vi "prueba_modbus.vi"() -> ()   [LabVIEW 2021, in "Test_VIs.lvlib"]
uses:
  Test_VIs.lvlib
  <vilib>/Modbus/master/Modbus Master.lvclass
  <vilib>/Modbus/master/Create Master Instance (TCP).vi
panel:
  out "ComunicacionCRIO":bool
  out "coil values":bool[](array[boolean])
  in  "stop":bool
  out "element":u16
  out "element 2":u16
  out "element 3":u16
  out "Array":sgl[](array[numeric])
  in  "coil values 2":bool[](array[boolean])
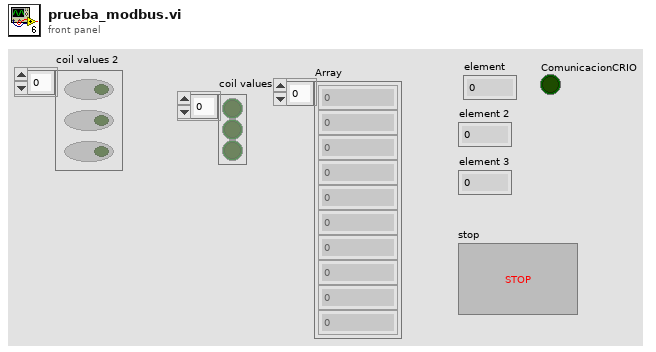
[diagram p1: front panel]
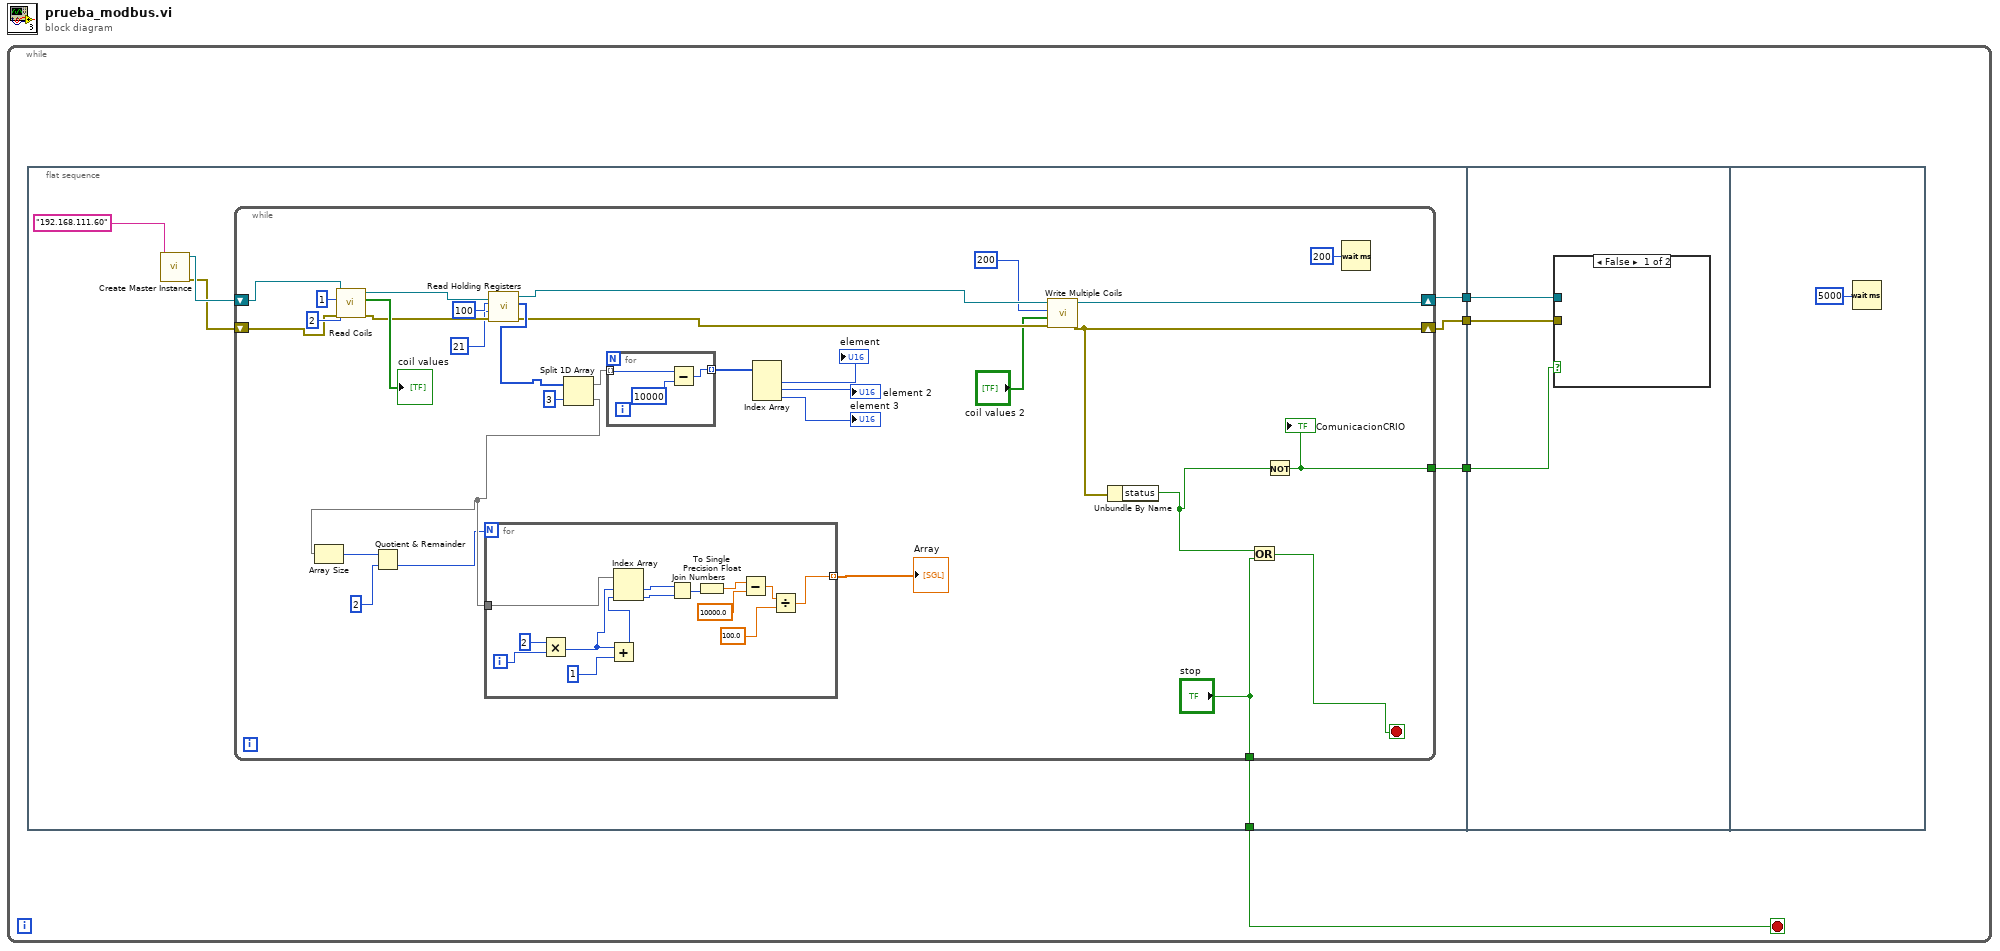
[diagram p0: block diagram]
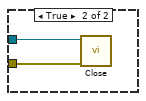
[diagram p2: hidden frame]
diagram:
  n1 = while {
    stop <- w1 stop-if-true
    n2 = flat-sequence {
      tunnel: [w8] -> w4
      tunnel: [w7] -> w3
      tunnel: [w6] -> w2
      tunnel: [w5] -> w1
      tunnel: w4 -> [w63]
      tunnel: w3 -> [w62]
      tunnel: w2 -> [w61]
      frame #0 {
        n3 = call-poly <vilib>:"Create Master Instance.vi"("address"="192.168.111.60") -> ("error out"=w9:errorcluster, "TCP master instance"=w10:refnum<class "Modbus Master.lvclass">)  [unwired: 9 in]
        n4 = while {
          shift-right: [w18] -> w7
          shift-left: w10 -> [w20]
          shift-right: [w17] -> w6
          shift-left: w9 -> [w19]
          tunnel: [w14] -> w8
          tunnel: ["stop"] -> w5
          stop <- w16 stop-if-true
          n5 = call-dynamic "Read Coils.vi"("error in (no error)"=w19, "number of coils"=u16 2, "starting address"=u16 1, "Modbus master in"=w20) -> ("error out"=w39:errorcluster, "coil values"=→"coil values":bool[], "Modbus master out"=w40:refnum<class "Modbus Master.lvclass">)  [unwired: 5 in]
          n6 = call-dynamic "Read Holding Registers.vi"("error in (no error)"=w39, "number of holding registers"=u16 21, "starting address"=u16 100, "Modbus master in"=w40) -> ("error out"=w23:errorcluster, "register values"=w27:u16[], "Modbus master out"=w24:refnum<class "Modbus Master.lvclass">)  [unwired: 5 in]
          n7 = Split 1D Array(array=w27, index=3) -> (first subarray=w26:u16[], second subarray=w32:u16[])
          n8 = Array Size(array=w32) -> (size(s)=w31:i32)
          n9 = Quotient & Remainder(x=w31, y=2) -> (floor(x/y)=w28:i32)  [unwired: 1 out]
          n10 = for {
            N: w28 -> [_]
            tunnel: w32 -> [w53]
            tunnel: [w50] -> w29 mode=indexing
            i -> [w60]
            n11 = Multiply(x=2, y=w60) -> (x*y=w58:i32)
            n12 = Add(x=w58, y=1) -> (x+y=w56:i32)
            n13 = Index Array(array=w53, index #1=w58, index #2=w56) -> (element #1=w55:u16, element #2=w54:u16)
            n14 = Join Numbers(hi=w55, lo=w54) -> ((hi.lo)=w52:u32)
            n15 = To Single Precision Float(number=w52) -> (single precision float=w49:sgl)
            n16 = Subtract(x=w49, y=sgl 10000.0) -> (x-y=w47:sgl)
            n17 = Divide(x=w47, y=sgl 100.0) -> (x/y=w50:sgl)
          }
          "Array" <- w29
          n18 = for {
            tunnel: w26 -> [w46] mode=indexing
            tunnel: [w44] -> w25 mode=indexing
            n19 = Subtract(x=w46, y=u16 10000) -> (x-y=w44:u16)
          }
          n20 = Index Array(array=w25) -> (element #1=→"element":u16, element #2=→"element 2":u16, element #3=→"element 3":u16)  [unwired: 3 in]
          n21 = call-dynamic "Write Multiple Coils.vi"("error in (no error)"=w23, "coil values"="coil values 2", "starting address"=u16 200, "Modbus master in"=w24) -> ("error out"=w17:errorcluster, "Modbus master out"=w18:refnum<class "Modbus Master.lvclass">)  [unwired: 6 in]
          n22 = Unbundle By Name(w17) -> ("status"=w15:bool)
          n23 = Or(x=w15, y="stop") -> (x .or. y?=w16:bool)
          n24 = Not(x=w15) -> (.not. x?=w14:bool)
          "ComunicacionCRIO" <- w14
          n25 = Wait (ms)(milliseconds to wait=u32 200) -> ()  [unwired: 1 out]
        }
      }
      frame #1 {
        n26 = case shown="False" w63 {
          tunnel: w62 -> [_ w65]
          tunnel: w61 -> [_ w64]
          frame False {
          }
          frame True {
            n27 = call-dynamic "Close.vi"("error in (no error)"=w64, "Modbus master in"=w65) -> ()  [unwired: 9 in, 1 out]
          }
        }
      }
      frame #2 {
        n28 = Wait (ms)(milliseconds to wait=u32 5000) -> ()  [unwired: 1 out]
      }
    }
  }
